vi "receiveData.vi"(8 "error in (no error)":errorcluster, 11 "Model in":refnum<class "Model.lvclass">) -> (0 "error out":errorcluster, 3 "Model out":refnum<class "Model.lvclass">)   [LabVIEW 2013, in "Model.lvclass"]
uses:
  Model.lvclass
  Model.lvclass/Model.ctl
  <userlib>/Common/ILC/ILC/ILC.lvclass
  UserEvents/UserEvents.lvclass
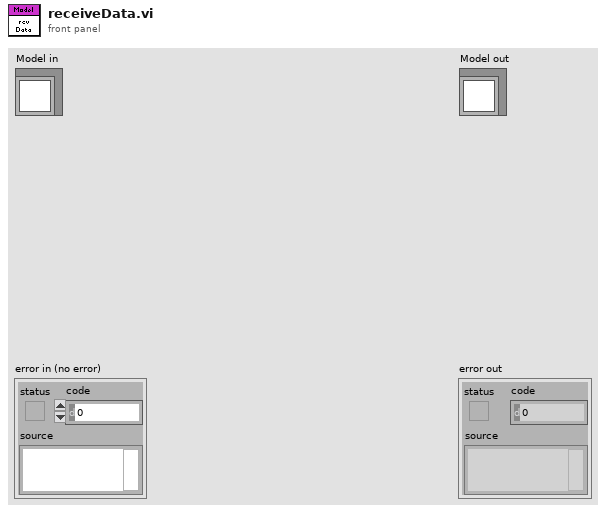
[diagram p1: front panel]
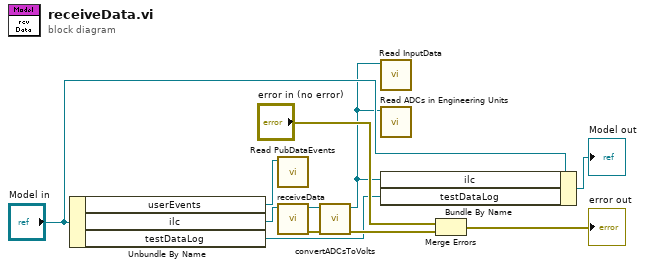
[diagram p0: block diagram]
diagram:
  n1 = Unbundle By Name("Model in") -> ("userEvents"=w5:refnum<class "UserEvents.lvclass">, "ilc"=w3:refnum<class "ILC.lvclass">, "testDataLog"=w1:refnum<class "TestDataLog.lvclass">)
  n2 = call "Read PubDataEvents.vi"("UserEvents in"=w5) -> ()  [unwired: 9 in, 2 out]
  n3 = call <userlib>:"receiveData.vi"("ILC in"=w3) -> ("error out"=w6:errorcluster, "ILC out"=w7:refnum<class "ILC.lvclass">)  [unwired: 9 in]
  n4 = call <userlib>:"convertADCsToVolts.vi"("error in (no error)"=w6, "ILC in"=w7) -> ("error out"=w2:errorcluster, "ILC out"=w4:refnum<class "ILC.lvclass">)  [unwired: 8 in]
  n5 = call <userlib>:"Read InputData.vi"("ILC in"=w4) -> ()  [unwired: 9 in, 2 out]
  n6 = call <userlib>:"Read ADCs in Engineering Units.vi"("ILC in"=w4) -> ()  [unwired: 9 in, 2 out]
  n7 = Bundle By Name(cluster="Model in", "ilc"=w4, "testDataLog"=w1) -> (→"Model out":refnum<class "Model.lvclass">)
  n8 = Merge Errors("error in (no error)", w2) -> (→"error out":errorcluster)
